vi "Type Specialization Structure - Lesson 2.vi"() -> ()   [LabVIEW 2023]
doc: "Lesson 2 shows how the <b>Assert Structural Type Match</b> and related assert VIs work with the <b>Type Specialization</b> structure."
uses:
  cc8e7cd3-c207-428c-844b-baa30fb5aa95.vi
  292d1115-d2ce-4442-b99f-0a58dd1bdec9.vi
  6a889f10-457d-4def-a7c0-5bf32b52c606.vi
  e5598f79-2995-40de-8c43-b4ddd0d8a5f5.vi
  718386fe-fd2c-47bf-8591-779b815879f1.vi
  cc8e7cd3-c207-428c-844b-baa30fb5aa95.vi/ff40df25-0e41-4205-825d-56c19dc320b6.vi
  6a889f10-457d-4def-a7c0-5bf32b52c606.vi/c19e8020-341a-4fad-8634-428a0c9ad438.vi
  e5598f79-2995-40de-8c43-b4ddd0d8a5f5.vi/ff40df25-0e41-4205-825d-56c19dc320b6.vi
  <vilib>/Array/Sort 2D Array - Pop Stack.vi
  <vilib>/Array/Sort 2D Array - Push Stack.vi
  718386fe-fd2c-47bf-8591-779b815879f1.vi/269d4b3b-47f5-49e3-8884-44851e4dd9d5.vi
  718386fe-fd2c-47bf-8591-779b815879f1.vi/6d99389c-673d-4efb-bf33-19b32bcf4cf8.vi
  6a889f10-457d-4def-a7c0-5bf32b52c606.vi/c19e8020-341a-4fad-8634-428a0c9ad438.vi/b30c0498-5c87-4a37-a7a8-8ea35c3fd313.vi
  <vilib>/Utility/Debug Log/Display.vi
panel:
  out "sorted 2D array":i32[][](array[numeric])
  # "Overview: This second lesson shows how the Assert Structural Type Match and related assert VIs work with the Type Specialization structure.\n\nInstructions: \n1. Open the block diagram of this VI. Review the lessons presented there.\n2. Run the VI to see the results."
  # "Rows were sorted by the value of the middle column."
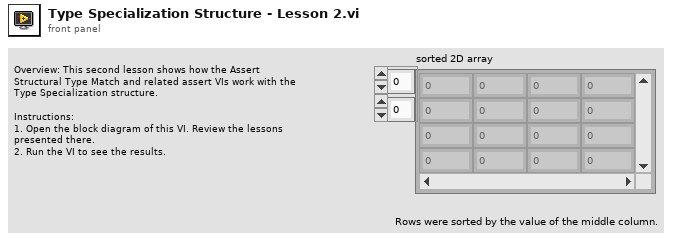
[diagram p1: front panel]
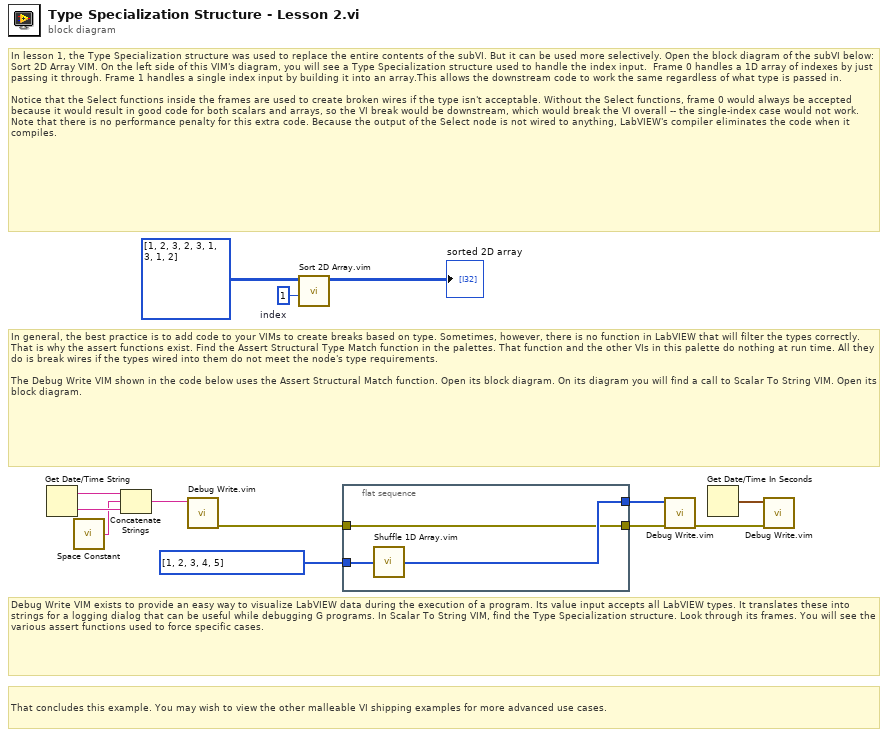
[diagram p0: block diagram]
diagram:
  w1 = 1  # index
  # "That concludes this example. You may wish to view the other malleable VI shipping examples for more advanced use cases."
  # "Debug Write VIM exists to provide an easy way to visualize LabVIEW data during the execution of a program. Its value input accepts all LabVIEW types. It translates these into strings for a logging dialog that can be useful while debugging G programs. In Scalar To String VIM, find the Type Specialization structure. Look through its frames. You will see the various assert functions used to force specific cases."
  # "In general, the best practice is to add code to your VIMs to create breaks based on type. Sometimes, however, there is no function in LabVIEW that will filter the types correctly. That is why the assert functions exist. Find the Assert Structural Type Match function in the palettes. That function and the other VIs in this palette do nothing at run time. All they do is break wires if the types wired into them do not meet the node's type requirements.\n\nThe Debug Write VIM shown in the code below uses the Assert Structural Match function. Open its block diagram. On its diagram you will find a call to Scalar To String VIM. Open its block diagram."
  # "In lesson 1, the Type Specialization structure was used to replace the entire contents of the subVI. But it can be used more selectively. Open the block diagram of the subVI below: Sort 2D Array VIM. On the left side of this VIM's diagram, you will see a Type Specialization structure used to handle the index input.  Frame 0 handles a 1D array of indexes by just passing it through. Frame 1 handles a single index input by building it into an array.This allows the downstream code to work the same regardless of what type is passed in. \n\nNotice that the Select functions inside the frames are used to create broken wires if the type isn't acceptable. Without the Select functions, frame 0 would always be accepted because it would result in good code for both scalars and arrays, so the VI break would be downstream, which would break the VI overall -- the single-index case would not work. Note that there is no performance penalty for this extra code. Because the output of the Select node is not wired to anything, LabVIEW's compiler eliminates the code when it compiles."
  n1 = Get Date/Time String() -> (date string=w11:string, time string=w10:string)  [unwired: 3 in]
  n2 = call <vilib>:"Space Constant.vi"() -> ("String"=w9:string)
  n3 = Concatenate Strings(w11, w9, w10) -> (w4:string)
  n4 = call "Debug Write.vim"("value"=w4) -> ("error out"=w6:errorcluster)  [unwired: 10 in]
  n5 = call "Sort 2D Array.vim"("index"=w1, "2D array"=i32[][] [[1, 2, 3], [2, 3, 1], [3, 1, 2]]) -> ("sorted 2D array"=→"sorted 2D array":i32[][])  [unwired: 8 in, 1 out]
  n6 = flat-sequence {
    tunnel: i32[] [1, 2, 3, 4, 5] -> [w16]
    tunnel: w6 -> [w14]
    tunnel: [w15] -> w5
    tunnel: [w14] -> w3
    frame #0 {
      n7 = call "Shuffle 1D Array.vim"("array"=w16) -> ("shuffled array"=w15:i32[])  [unwired: 4 in]
    }
  }
  n8 = call "Debug Write.vim"("error in (no error)"=w3, "value"=w5) -> ("error out"=w8:errorcluster)  [unwired: 9 in]
  n9 = Get Date/Time In Seconds() -> (seconds since 1Jan1904=w7:timestamp)
  n10 = call "Debug Write.vim"("error in (no error)"=w8, "value"=w7) -> ()  [unwired: 9 in, 1 out]
